vi "Queues FGV.vi"(8 "error in":errorcluster, 11 "Action":T1) -> (0 "error out":errorcluster, 3 "Queues Out":T2)   [LabVIEW 2024, in "ECU InterComm.lvlib"]
uses:
  ECU InterComm.lvlib
  QMH Item.ctl
  Process Queues.ctl
  General Actions.ctl
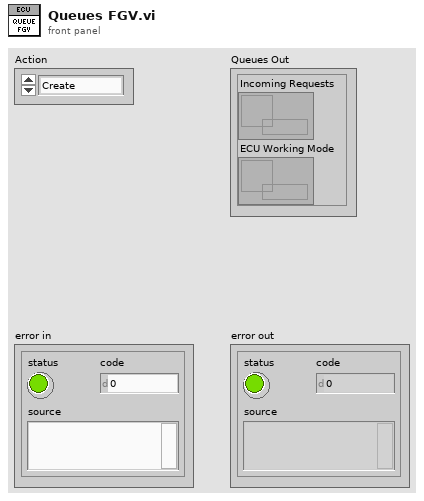
[diagram p1: front panel]
types:
  T1 = typedef "ECU InterComm.lvlib/General Actions.ctl" = enum16{"Create", "Get", "Destroy"}
  T2 = typedef "ECU InterComm.lvlib/Process Queues.ctl" = cluster{"Incoming Requests":refnum<queue>, "ECU Working Mode":refnum<queue>}
  T3 = typedef "ECU InterComm.lvlib/QMH Item.ctl" = cluster{"Message":string, "Data":variant}
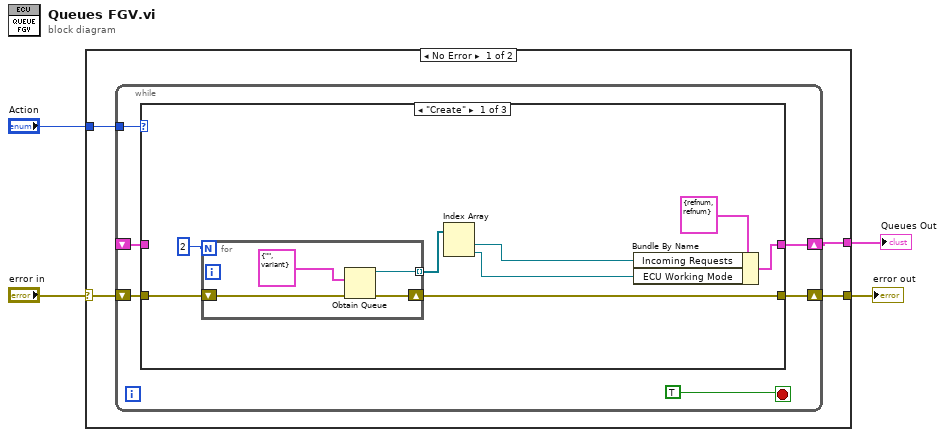
[diagram p0: block diagram]
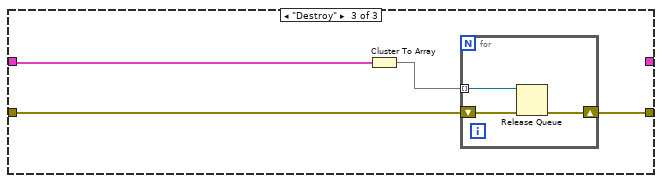
[diagram p3: hidden frame]
diagram:
  n1 = case shown="No Error" "error in" {
    selector: "error in" -> [w5 w36]
    tunnel: "Action" -> [w8 _]
    tunnel: [w7 w36] -> w3
    tunnel: [w6 _] -> w2
    frame No Error {
      n2 = while {
        tunnel: w8 -> [w13]
        shift-right: [w12] -> w7
        shift-left: w5 -> [w11]
        shift-right: [w10] -> w6
        shift-left: _ -> [w9]
        stop <- TRUE stop-if-true
        n3 = case shown="\"Create\"" w13 {
          tunnel: [w18 w28 w32] -> w12
          tunnel: w11 -> [w17 w28 w31]
          tunnel: [w21 w27 _] -> w10
          tunnel: w9 -> [_ w27 w29]
          frame "Create" {
            n4 = for {
              N: 2 -> [_]
              shift-right: [w25] -> w18
              shift-left: w17 -> [w26]
              tunnel: [w23] -> w20 mode=indexing
              n5 = Obtain Queue(element data type=T3 {"Message"="", "Data"=variant}, error in (no error)=w26) -> (queue out=w23:refnum<queue>, error out=w25:errorcluster)  [unwired: 3 in, 1 out]
            }
            n6 = Index Array(array=w20) -> (element #1=w15:refnum<queue>, element #2=w16:refnum<queue>)  [unwired: 2 in]
            n7 = Bundle By Name(cluster=T2 {"Incoming Requests"=refnum, "ECU Working Mode"=refnum}, "Incoming Requests"=w15, "ECU Working Mode"=w16) -> (w21:T2)
          }
          frame "Get", Default {
          }
          frame "Destroy" {
            n8 = Cluster To Array(cluster=w29) -> (array=w30:refnum<queue>[])
            n9 = for {
              shift-right: [w34] -> w32
              shift-left: w31 -> [w35]
              tunnel: w30 -> [w33] mode=indexing
              n10 = Release Queue(queue=w33, error in (no error)=w35) -> (error out=w34:errorcluster)  [unwired: 1 in, 2 out]
            }
          }
        }
      }
    }
    frame Error {
    }
  }
  "error out" <- w3
  "Queues Out" <- w2
